vi "Ex7_LocalVariables.vi"() -> ()   [LabVIEW 2024]
panel:
  out "0-100":dbl
  out "0-1":dbl
  in  "stop":bool
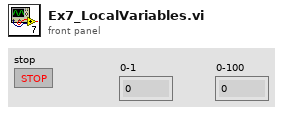
[diagram p1: front panel]
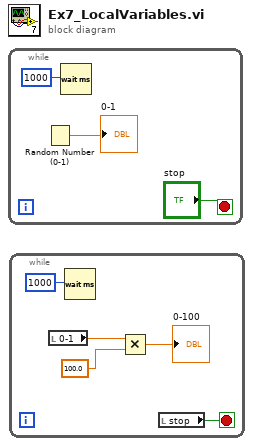
[diagram p0: block diagram]
diagram:
  n1 = while {
    stop <- "stop" stop-if-true
    n2 = Random Number (0-1)() -> (number: 0 to 1=→"0-1":dbl)
    n3 = Wait (ms)(milliseconds to wait=1000) -> ()  [unwired: 1 out]
  }
  n4 = while {
    stop <- w7 stop-if-true
    n5 = local read "0-1"() -> (w6:dbl)
    n6 = Wait (ms)(milliseconds to wait=1000) -> ()  [unwired: 1 out]
    n7 = Multiply(x=w6, y=100.0) -> (x*y=→"0-100":dbl)
    n8 = local read "stop"() -> (w7:bool)
  }
